vi "Untitled 32.vi"   [LabVIEW 2014]
uses:
  <vilib>/FPGAPlugInAG/cRIO-9063/niLvFpga_Open_cRIO-9063.vi
  <vilib>/rvi/interface/common/dynamic/niFpgaDynamicAddResources.vi
  <vilib>/FPGAPlugInAG/Dynamic/niLvFpga_Close_Dynamic.vi
  <vilib>/rvi/interface/nirviOpenFPGA/nirviOpenFPGA.xnode
  akhil3/FPGA Bitfiles/trailswithgps_FPGATarget_recursiveakhil_QexfQQGvF84.lvbitx
  recursive akhil.vi
  <vilib>/rvi/interface/nirviCloseFPGA/nirviCloseFPGA.xnode
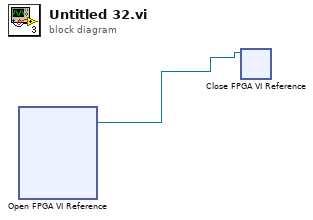
[diagram p0: block diagram]
diagram:
  n1 = xnode "Open FPGA VI Reference"() -> ("FPGA VI Reference Out"=w1:refnum<k20>)  [unwired: 2 in, 1 out]
  n2 = xnode "Close FPGA VI Reference"("FPGA VI Reference In"=w1) -> ()  [unwired: 1 in, 1 out]
